vi "server_2nd_try.vi"() -> ()   [LabVIEW 2012]
panel:
  out "record":T1
  out "setting":u32
  out "done":bool
  out "?":T2
  out "Settings":T3(array[cluster])
  out "?":T4(ring)
  out "packet data":T2
  in  "Stop":bool
  out "server ID":u32
  out "welcome message":string
  in  "manager":T5={"address"="localhost", "port"=7682, "password"=""}
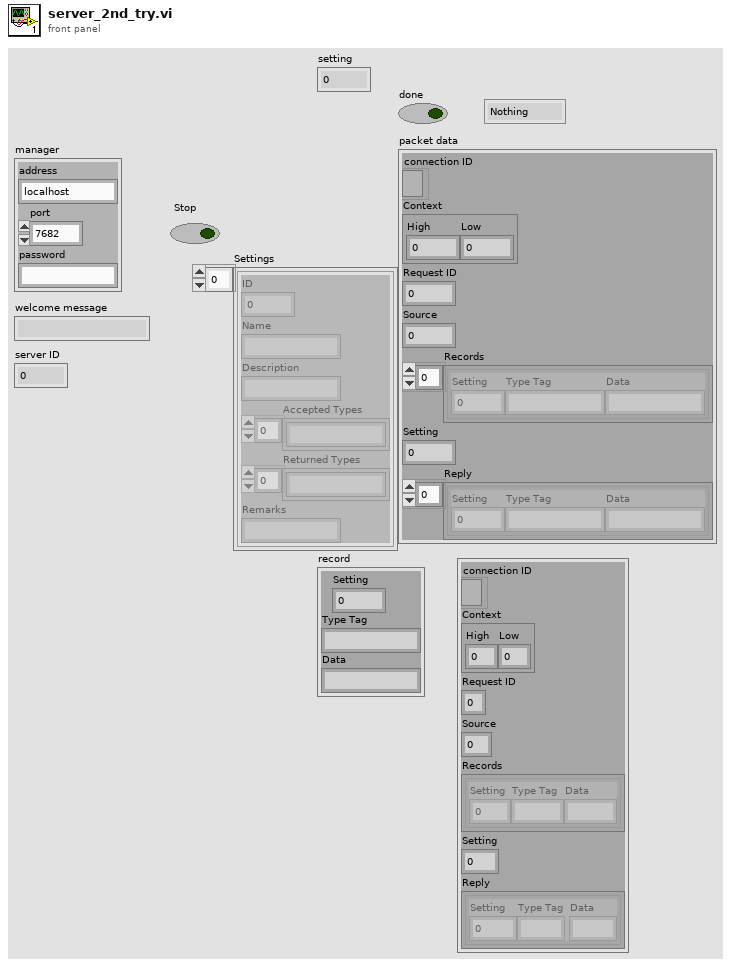
[diagram p1: front panel]
types:
  T1 = cluster{"Setting":u32, "Type Tag":string, "Data":string}
  T2 = cluster{"connection ID":refnum<k5>, "Context":cluster{"High":u32, "Low":u32}, "Request ID":i32, "Source":u32, "Records":cluster{"Setting":u32, "Type Tag":string, "Data":string}[], "Setting":u32, "Reply":cluster{"Setting":u32, "Type Tag":string, "Data":string}[]}
  T3 = cluster{"ID":u32, "Name":string, "Description":string, "Accepted Types":string[], "Returned Types":string[], "Remarks":string}[]
  T4 = enum16{"Nothing", "Message", "Request", "Error", "Expire", "Expire All"}
  T5 = cluster{"address":string, "port":u16, "password":string}
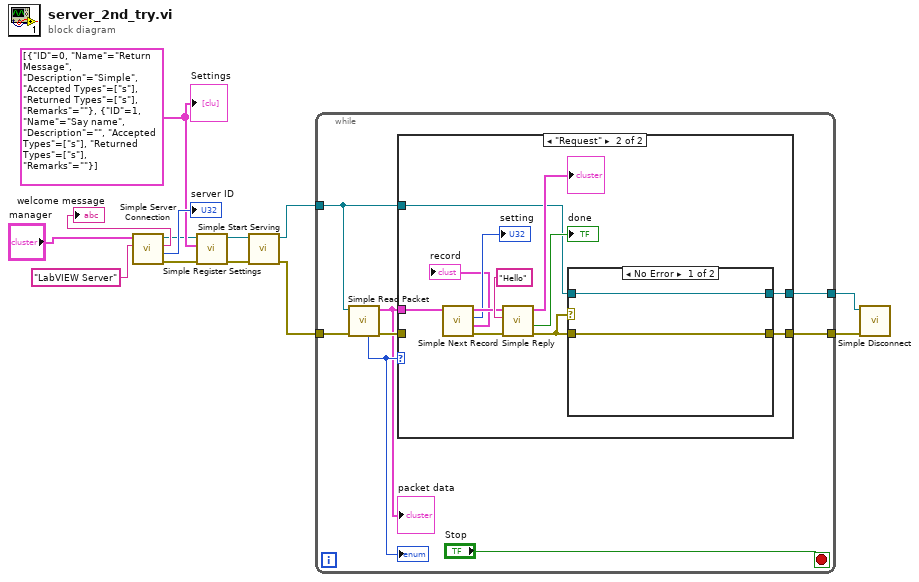
[diagram p0: block diagram]
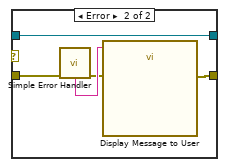
[diagram p3: hidden frame]
diagram:
  w7 = T3 [{"ID"=0, "Name"="Return Message", "Description"="Simple", "Accepted Types"=["s"], "Returned Types"=["s"], "Remarks"=""}, {"ID"=1, "Name"="Say name", "Description"="", "Accepted Types"=["s"], "Returned Types"=["s"], "Remarks"=""}] ("Settings")
  n1 = call <userlib>:"Simple Server Connection.vi"("connection name (LabVIEW Server)"="LabVIEW Server", "manager"="manager") -> ("error out"=w6:errorcluster, "server ID"=→"server ID":u32, "welcome message"=→"welcome message":string, "connection ID out"=w5:refnum<k5>)  [unwired: 2 in]
  n2 = call <userlib>:"Simple Register Settings.vi"("error in (no error)"=w6, "Settings"=w7, "connection ID"=w5) -> ("error out"=w3:errorcluster, "connection ID out"=w4:refnum<k5>)  [unwired: 3 in]
  n3 = call <userlib>:"Simple Start Serving.vi"("error in (no error)"=w3, "connection ID"=w4) -> ("error out"=w1:errorcluster, "connection ID out"=w2:refnum<k5>)  [unwired: 4 in]
  n4 = while {
    tunnel: [w15] -> w9
    tunnel: [w17] -> w8
    tunnel: w1 -> [w20]
    tunnel: w2 -> [w16]
    stop <- "Stop" stop-if-true
    n5 = call <userlib>:"Simple Read Packet.vi"("connection ID"=w16, "error in (no error)"=w20) -> ("result"=w19:T4, "packet data"=w14:T2, "error out"=w18:errorcluster)  [unwired: 3 in, 2 out]
    "packet data" <- w14
    "?" <- w19
    n6 = case shown="\"Request\"" w19 {
      tunnel: w18 -> [w23 _]
      tunnel: [w23 w31] -> w17
      tunnel: w16 -> [w22 w30]
      tunnel: [w22 w29] -> w15
      tunnel: w14 -> [_ w28]
      frame "Nothing", Default {
      }
      frame "Request" {
        n7 = call <userlib>:"Simple Next Record.vi"("packet data"=w28) -> ("packet data out"=w27:T2, "setting"=→"setting":u32, "record"=→"record":T1, "error out"=w26:errorcluster)  [unwired: 4 in, 1 out]
        n8 = call <userlib>:"Simple Reply.vi"("error in (no error)"=w26, "data"="Hello", "packet data"=w27) -> ("error out"=w32:errorcluster, "done"=→"done":bool, "packet data out"=→"?":T2)  [unwired: 2 in]
        n9 = case shown="No Error" w32 {
          tunnel: w32 -> [w37 w42]
          tunnel: [w37 w39] -> w31
          tunnel: w30 -> [w36 w38]
          tunnel: [w36 w38] -> w29
          frame No Error {
          }
          frame Error {
            n10 = call <vilib>:"Simple Error Handler.vi"("error in (no error)"=w42) -> ("error out"=w40:errorcluster, "message"=w41:string)  [unwired: 4 in, 3 out]
            n11 = call "Display Message to User"("error in (no error)"=w40, "Message"=w41) -> ("error out"=w39:errorcluster)  [unwired: 8 in, 1 out]
          }
        }
      }
    }
  }
  n12 = call <userlib>:"Simple Disconnect.vi"("error in (no error)"=w8, "connection ID"=w9) -> ()  [unwired: 5 in, 1 out]
  "Settings" <- w7
